vi "Status ProgramInfo.vi"(7 "Pattern No. (-1:All)":i32=-1, 8 "error in (no error)":errorcluster, 10 "Address (0)":i32, 11 "VISA resource name":refnum<visa-resource-name>) -> (0 "error out":errorcluster, 1 "pattern numbers":i32[](array[numeric]), 2 "#program patterns":i32, 3 "VISA resource name out":refnum<visa-resource-name>, 4 "Write date":dbl format="%<%Y/%m/%d>T", 5 "Pattern Name":string)   [LabVIEW 2016, in "Environment Chamber.lvlib" / "Climatic Chamber.lvlib"]
doc: "<b>Program pattern usage monitor</B>\n\nReturns the program pattern information with set date (Pattern No.: -1) or\nReturns the pattern number of the specified program pattern and the write date (Pattern No.: X)."
uses:
  Climatic Chamber.lvlib
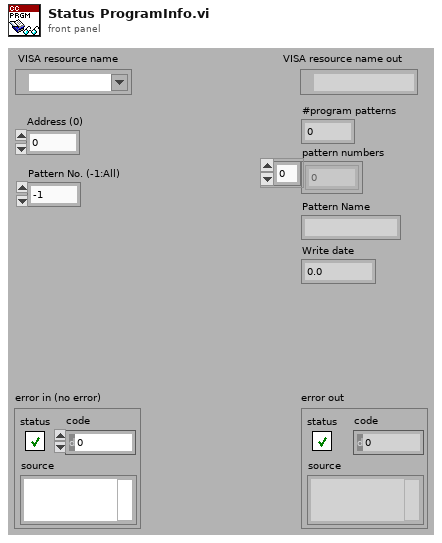
[diagram p1: front panel]
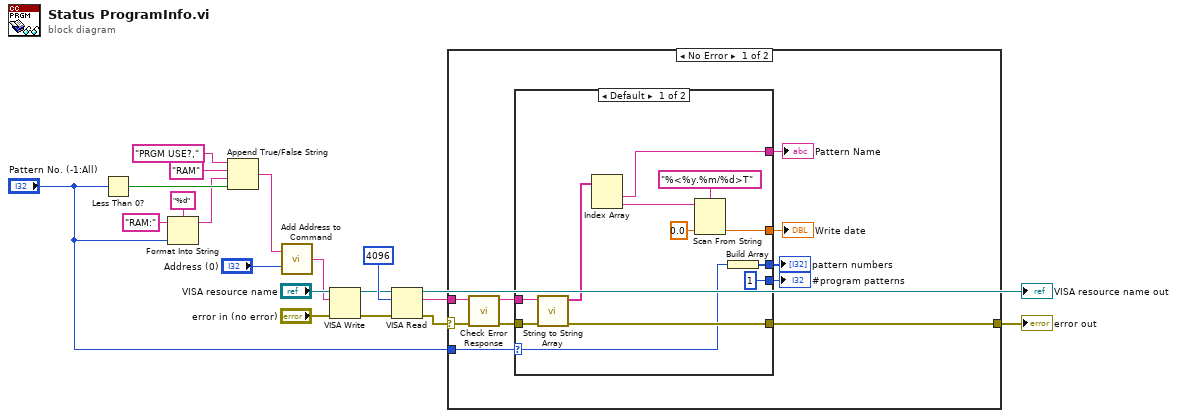
[diagram p0: block diagram]
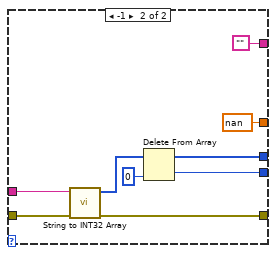
[diagram p2: hidden frame]
diagram:
  n1 = Less Than 0?(x="Pattern No. (-1:All)") -> (x < 0?=w2:bool)
  n2 = Format Into String(format string="%d", initial string="RAM:", "Pattern No. (-1:All)") -> (resulting string=w1:string)  [unwired: 1 in, 1 out]
  n3 = Append True/False String(1:w2, 2:w1, 3:"RAM" ("true string"), 4:"PRGM USE?,") -> (0:w4:string)
  n4 = call "Add Address to Command.vi"("Address (0)"="Address (0)", "Command"=w4) -> ("Command OUT"=w13:string)
  n5 = VISA Write(VISA resource name="VISA resource name", write buffer=w13, error in (no error)="error in (no error)") -> (VISA resource name out=w16:refnum<visa-resource-name>, error out=w15:errorcluster)  [unwired: 1 out]
  n6 = VISA Read(VISA resource name=w16, byte count=u32 4096, error in (no error)=w15) -> (VISA resource name out=→"VISA resource name out":refnum<visa-resource-name>, read buffer=w11:string, error out=w12:errorcluster)  [unwired: 1 out]
  n7 = case shown="No Error" w12 {
    selector: w12 -> [w28 w51]
    tunnel: w11 -> [w29 _]
    tunnel: [w26 w51] -> w10
    tunnel: "Pattern No. (-1:All)" -> [w22 _]
    frame No Error {
      n8 = call "Check Error Response.vi"("error in (no error)"=w28, "read String"=w29) -> ("error out"=w27:errorcluster, "String out"=w25:string)  [unwired: 7 in, 1 out]
      n9 = case shown="Default" w22 {
        selector: w22 -> [w38 _]
        tunnel: w27 -> [w40 w50]
        tunnel: [w39 w49] -> w26
        tunnel: w25 -> [w41 w48]
        tunnel: [1 w45] -> w24
        tunnel: [w37 w44] -> w23
        tunnel: [w32 nan] -> w21
        tunnel: [w31 ""] -> w20
        frame Default {
          n10 = call "String to String Array.vi"("error in (no error)"=w40, "String received"=w41) -> ("error out"=w39:errorcluster, "Array Data"=w36:string[])  [unwired: 8 in]
          n11 = Index Array(array=w36) -> (element #1=w31:string, element #2=w33:string)  [unwired: 2 in]
          n12 = Scan From String(format string="%<%y.%m/%d>T", input string=w33, default 1=0.0) -> (output 1=w32:dbl)  [unwired: 2 in, 3 out]
          n13 = Build Array(w38) -> (w37:i32[])
        }
        frame -1 {
          n14 = call "String to INT32 Array.vi"("error in (no error)"=w50, "String received"=w48) -> ("error out"=w49:errorcluster, "Array Data"=w47:i32[])  [unwired: 8 in]
          n15 = Delete From Array(array=w47, index=0) -> (deleted portion=w45:i32, array with subset deleted=w44:i32[])  [unwired: 1 in]
        }
      }
      "#program patterns" <- w24
      "pattern numbers" <- w23
      "Write date" <- w21
      "Pattern Name" <- w20
    }
    frame Error {
    }
  }
  "error out" <- w10
